vi "inputTwoEntry.vi"(9 "inputFilePath":path=path "G:/Document/랩타임측정시스템/Program/CommonResource/EVEntry.txt") -> (0 "ErrorOutput":errorcluster, 2 "OutputData":T1(array[cluster]), 4 "StopButtonOutput":bool, 6 "OKButtonOutput":bool)   [LabVIEW 2020]
uses:
  <vilib>/Utility/file.llb/Read Delimited Spreadsheet (string).vi
panel:
  in  "DNFEntry-B":bool
  in  "DNFEntry-A":bool
  out "CurrentData-B":T2
  in  "InputEntry-B":i32
  out "CurrentData-A":T3
  in  "InputEntry-A":i32
  in  "Stop Button":bool
  in  "OK Button":bool
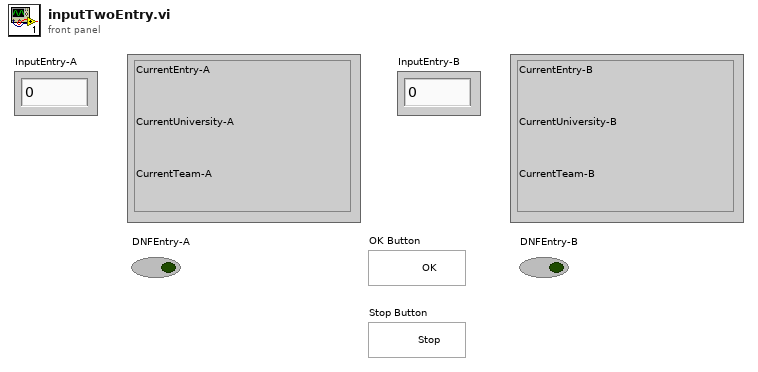
[diagram p1: front panel]
types:
  T1 = cluster{"CurrentEntry":string, "CurrentUniv":string, "CurrentTeam":string, "DNF":bool}[]
  T2 = cluster{"CurrentEntry-B":string, "CurrentUniversity-B":string, "CurrentTeam-B":string}
  T3 = cluster{"CurrentEntry-A":string, "CurrentUniversity-A":string, "CurrentTeam-A":string}
  T4 = enum16{"open", "replace", "create", "open or create", "replace or create", "replace or create with confirmation"}
  T5 = cluster{"CurrentEntry":string, "CurrentUniv":string, "CurrentTeam":string}
  T6 = cluster{"CurrentEntry":string, "CurrentUniv":string, "CurrentTeam":string, "DNF":bool}
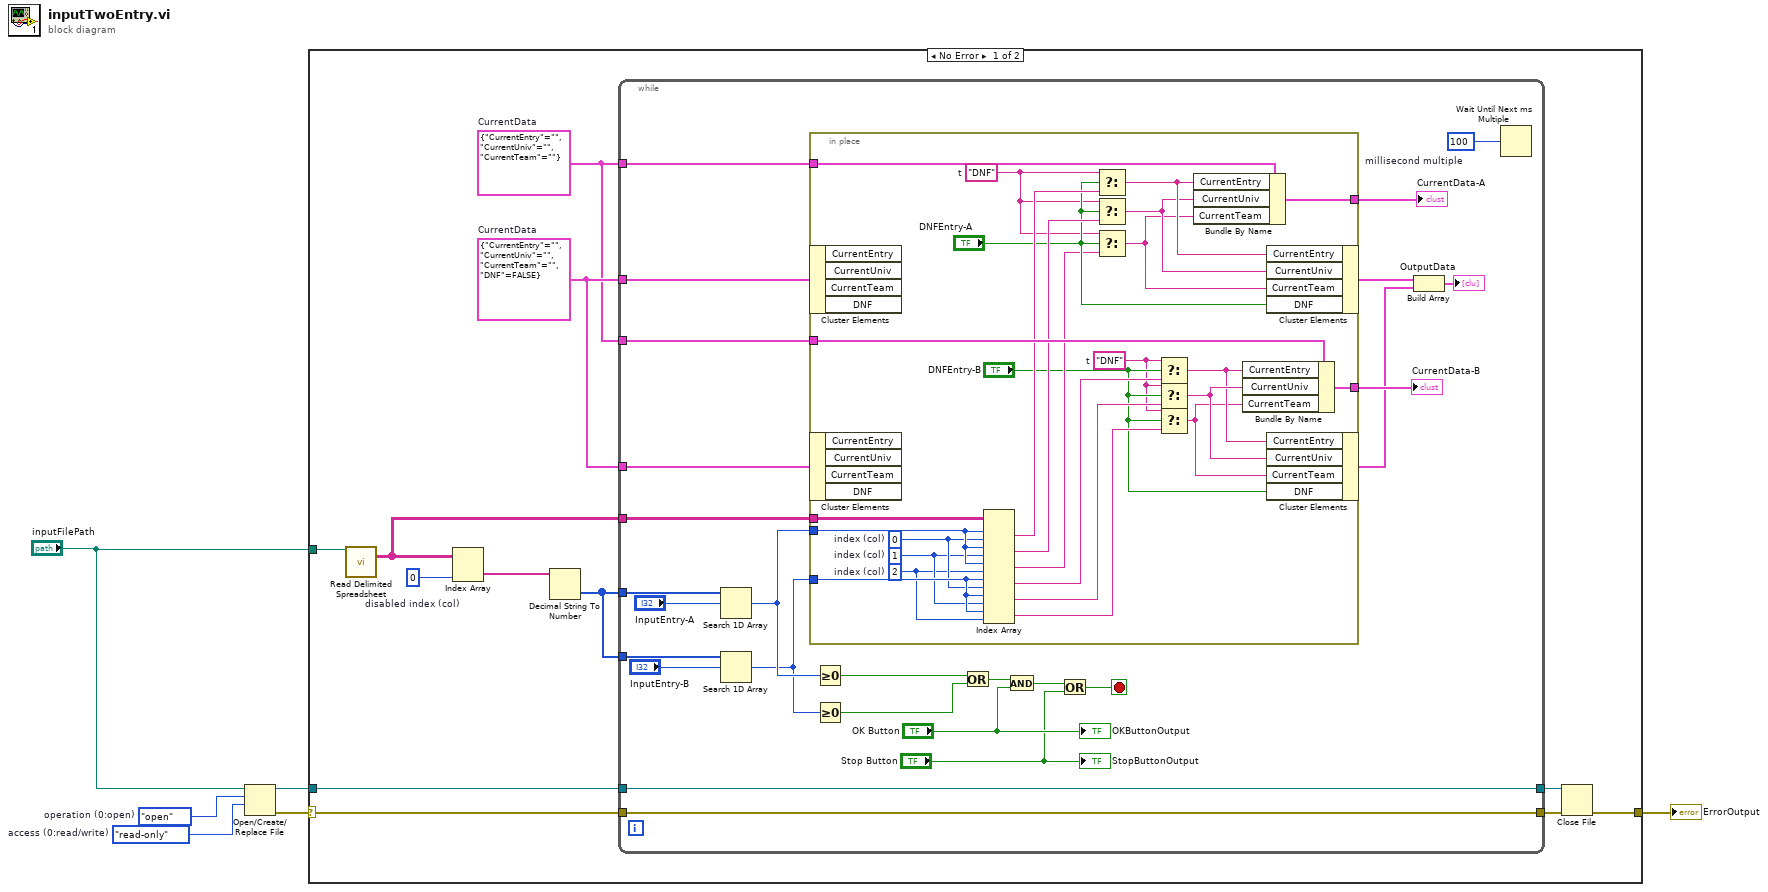
[diagram p0: block diagram]
diagram:
  w1 = enum16{"read/write", "read-only", "write-only"}."read-only"  # access (0:read/write)
  w3 = T4."open"  # operation (0:open)
  n1 = Open/Create/Replace File(file path (use dialog)="inputFilePath", operation (0:open)=w3, access (0:read/write)=w1) -> (refnum out=w2:refnum<file>, error out=w6:errorcluster)  [unwired: 3 in, 1 out]
  n2 = case shown="No Error" w6 {
    selector: w6 -> [w10 w71]
    tunnel: [w14 w71] -> w5
    tunnel: "inputFilePath" -> [w17 _]
    tunnel: w2 -> [w12 _]
    frame No Error {
      w7 = T5 {"CurrentEntry"="", "CurrentUniv"="", "CurrentTeam"=""}  # CurrentData
      w15 = 0  # disabled index (col)
      w8 = T6 {"CurrentEntry"="", "CurrentUniv"="", "CurrentTeam"="", "DNF"=FALSE}  # CurrentData
      n3 = call-poly <vilib>:"Read Delimited Spreadsheet.vi"("file path (dialog if empty)"=w17) -> ("all rows"=w16:string[][])  [unwired: 9 in, 5 out]
      n4 = Index Array "Index Array"(array=w16, index (col)=w15) -> (element=w18:string[])  [unwired: 1 in]
      n5 = Decimal String To Number(string=w18) -> (number=w9:i32[])  [unwired: 2 in, 1 out]
      n6 = while {
        tunnel: w9 -> [w44]
        tunnel: w16 -> [w43]
        tunnel: w8 -> [w40]
        tunnel: [w42] -> w13
        tunnel: w12 -> [w42]
        tunnel: [w41] -> w11
        tunnel: w10 -> [w41]
        tunnel: w9 -> [w38]
        tunnel: w8 -> [w37]
        tunnel: w7 -> [w22]
        tunnel: w7 -> [w19]
        stop <- w29 stop-if-true
        w39 = u32 100  # millisecond multiple
        n7 = Search 1D Array(1D array=w44, element="InputEntry-A") -> (index of element=w26:i32)  [unwired: 1 in]
        n8 = Search 1D Array(1D array=w38, element="InputEntry-B") -> (index of element=w25:i32)  [unwired: 1 in]
        n9 = in-place {
          in-place-border: w43 -> [w70]
          in-place-border: w26 -> [w69]
          in-place-border: w25 -> [w68]
          in-place-border: [w64] -> w23
          in-place-border: w22 -> [w63]
          in-place-border: w19 -> [w62]
          in-place-border: [w61] -> w21
          w45 = "DNF"  # t
          w56 = "DNF"  # t
          w65 = 2  # index (col)
          w66 = 1  # index (col)
          w67 = 0  # index (col)
          n10 = in-place-cluster #1(w40) -> ()  [unwired: 4 out]
          n11 = in-place-cluster #2(w37) -> ()  [unwired: 4 out]
          n12 = Index Array "Index Array"(array=w70, index (row) #1=w69, index (col) #1=w67, index (row) #2=w69, index (col) #2=w66, index (row) #3=w69, index (col) #3=w65, index (row) #4=w68, index (col) #4=w67, index (row) #5=w68, index (col) #5=w66, index (row) #6=w68, index (col) #6=w65) -> (element #1=w60:string, element #2=w58:string, element #3=w53:string, element #4=w52:string, element #5=w51:string, element #6=w50:string)
          n13 = Select(t=w56, s="DNFEntry-A", f=w60) -> (s? t:f=w59:string)
          n14 = Select(t=w56, s="DNFEntry-A", f=w58) -> (s? t:f=w55:string)
          n15 = Select(t=w56, s="DNFEntry-A", f=w53) -> (s? t:f=w54:string)
          n16 = Select(t=w45, s="DNFEntry-B", f=w52) -> (s? t:f=w48:string)
          n17 = Select(t=w45, s="DNFEntry-B", f=w51) -> (s? t:f=w49:string)
          n18 = Select(t=w45, s="DNFEntry-B", f=w50) -> (s? t:f=w47:string)
          n19 = Bundle By Name(cluster=w63, "CurrentEntry"=w59, "CurrentUniv"=w55, "CurrentTeam"=w54) -> (w64:T5)
          n20 = Bundle By Name(cluster=w62, "CurrentEntry"=w48, "CurrentUniv"=w49, "CurrentTeam"=w47) -> (w61:T5)
          n21 = in-place-cluster #1("CurrentEntry"=w59, "CurrentUniv"=w55, "CurrentTeam"=w54, "DNF"="DNFEntry-A") -> (w36:T6)
          n22 = in-place-cluster #2("CurrentEntry"=w48, "CurrentUniv"=w49, "CurrentTeam"=w47, "DNF"="DNFEntry-B") -> (w20:T6)
        }
        "CurrentData-A" <- w23
        "CurrentData-B" <- w21
        n23 = Greater Or Equal To 0?(x=w26) -> (x >= 0?=w35:bool)
        n24 = Greater Or Equal To 0?(x=w25) -> (x >= 0?=w34:bool)
        n25 = Or(x=w35, y=w34) -> (x .or. y?=w33:bool)
        n26 = And(x=w33, y="OK Button") -> (x .and. y?=w31:bool)
        n27 = Or(x=w31, y="Stop Button") -> (x .or. y?=w29:bool)
        n28 = Build Array "Build Array"(w36, w20) -> (→"OutputData":T1)
        n29 = Wait Until Next ms Multiple(millisecond multiple=w39) -> ()  [unwired: 1 out]
        "OKButtonOutput" <- "OK Button"
        "StopButtonOutput" <- "Stop Button"
      }
      n30 = Close File(refnum=w13, error in=w11) -> (error out=w14:errorcluster)  [unwired: 1 out]
    }
    frame Error {
    }
  }
  "ErrorOutput" <- w5
